vi "Clear Reading Buffer Data.vi"(8 "error in (no error)":errorcluster, 9 "Reading Buffer (smua.nvbuffer1)":string="smua.nvbuffer1", 10 "Data Type (0: Buffer Data)":i32(ring) items=["Buffer Data", "Cache Data"], 11 "VISA resource name":refnum<visa-resource-name>) -> (0 "error out":errorcluster, 3 "VISA resource name out":refnum<visa-resource-name>)   [LabVIEW 2019, in "Keithley 2600 Series.lvlib"]
doc: "Clears the reading buffer data or cache data."
uses:
  Keithley 2600 Series.lvlib
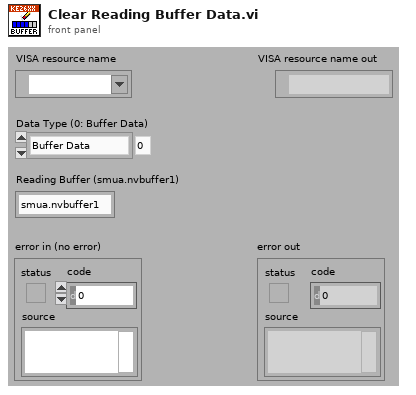
[diagram p1: front panel]
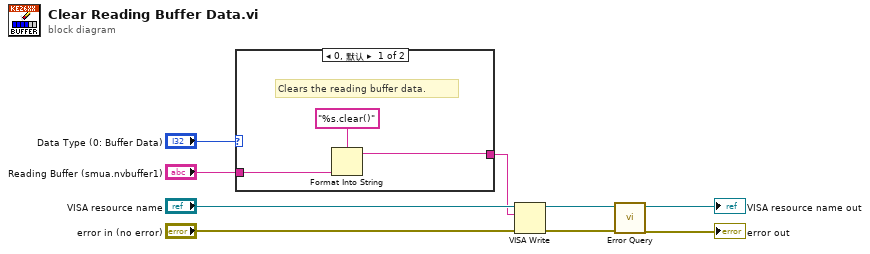
[diagram p0: block diagram]
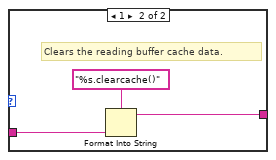
[diagram p2: hidden frame]
diagram:
  n1 = case shown="0, 默认" "Data Type (0: Buffer Data)" {
    tunnel: "Reading Buffer (smua.nvbuffer1)" -> [w11 w14]
    tunnel: [w10 w13] -> w1
    frame 0, Default {
      # "Clears the reading buffer data."
      n2 = Format Into String(format string="%s.clear()", w11) -> (resulting string=w10:string)  [unwired: 2 in, 1 out]
    }
    frame 1 {
      # "Clears the reading buffer cache data."
      n3 = Format Into String(format string="%s.clearcache()", w14) -> (resulting string=w13:string)  [unwired: 2 in, 1 out]
    }
  }
  n4 = VISA Write(VISA resource name="VISA resource name", write buffer=w1, error in (no error)="error in (no error)") -> (VISA resource name out=w7:refnum<visa-resource-name>, error out=w6:errorcluster)  [unwired: 1 out]
  n5 = call "Error Query.vi"("error in (no error)"=w6, "VISA resource name"=w7) -> ("error out"=→"error out":errorcluster, "VISA resource name out"=→"VISA resource name out":refnum<visa-resource-name>)  [unwired: 6 in, 2 out]
